vi "fb_lin_gain.vi"(7 "Kp":dbl, 8 "error in (no error)":errorcluster, 9 "V_in":dbl, 10 "w_d":dbl, 11 "w":dbl) -> (0 "error out":errorcluster, 2 "u_comps":dbl[](array[numeric]), 3 "u":dbl)   [LabVIEW 2019]
panel:
  out "u_l":dbl
  out "u_fbl":dbl
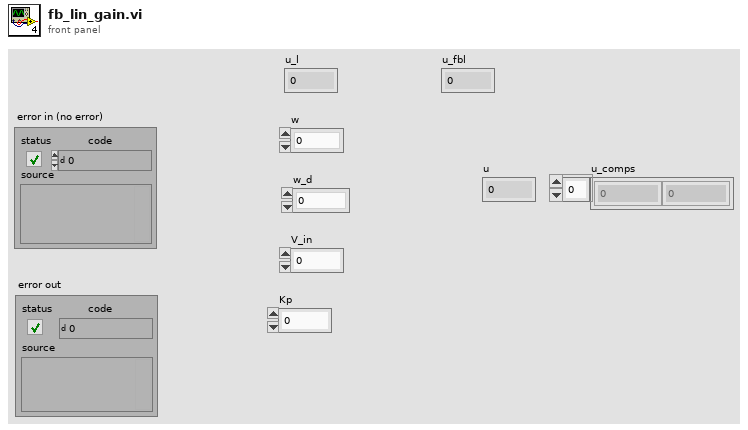
[diagram p1: front panel]
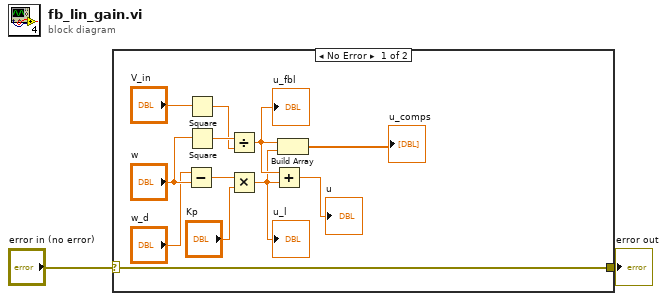
[diagram p0: block diagram]
diagram:
  n1 = case shown="No Error" "error in (no error)" {
    selector: "error in (no error)" -> [w4 w15]
    tunnel: [w4 w15] -> w2
    frame No Error {
      n2 = Subtract(x="w_d", y="w") -> (x-y=w6:dbl)
      n3 = Square(x="V_in") -> (x^2=w9:dbl)
      n4 = Square(x="w") -> (x^2=w14:dbl)
      n5 = Divide(x=w14, y=w9) -> (x/y=w12:dbl)
      "u_fbl" <- w12
      n6 = Multiply(x=w6, y="Kp") -> (x*y=w5:dbl)
      "u_l" <- w5
      n7 = Add(x=w12, y=w5) -> (x+y=→"u":dbl)
      n8 = Build Array(w12, w5) -> (→"u_comps":dbl[])
    }
    frame Error {
    }
  }
  "error out" <- w2
